vi "Read LINX I2C.vi"(8 "error in (no error)":errorcluster, 11 "TCS3472 in":refnum<class "TCS3472.lvclass">) -> (0 "error out":errorcluster, 2 "LINX I2C":refnum<class "LINX I2C.lvclass">, 3 "TCS3472 out":refnum<class "TCS3472.lvclass">)   [LabVIEW 2020, in "TCS3472.lvclass"]
uses:
  TCS3472.lvclass
  LINX I2C/LINX I2C.lvclass
  TCS3472.lvclass/TCS3472.ctl
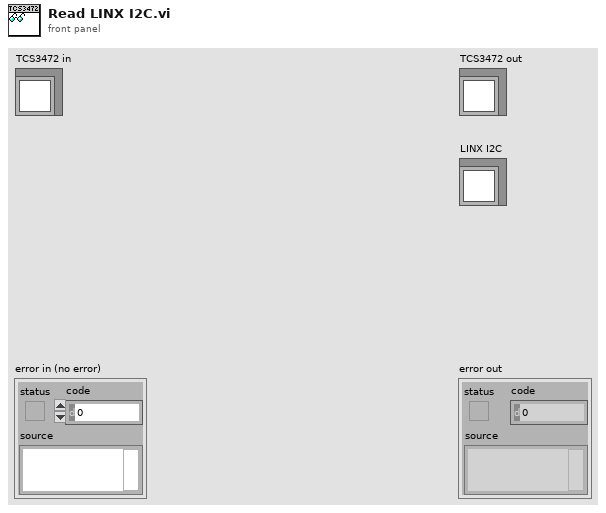
[diagram p1: front panel]
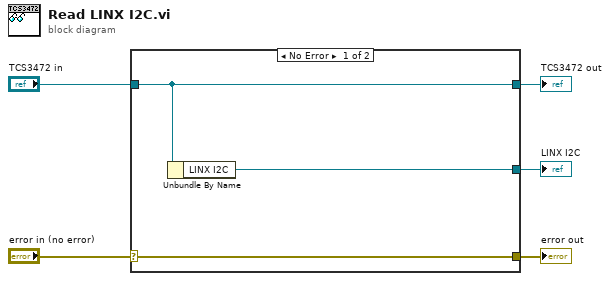
[diagram p0: block diagram]
diagram:
  n1 = case shown="No Error" "error in (no error)" {
    selector: "error in (no error)" -> [w8 w9]
    tunnel: [w8 w9] -> w4
    tunnel: [w7 w10] -> w2
    tunnel: "TCS3472 in" -> [w7 w10]
    tunnel: [w6 _] -> w1
    frame No Error {
      n2 = Unbundle By Name(w7) -> ("LINX I2C"=w6:refnum<class "LINX I2C.lvclass">)
    }
    frame Error {
    }
  }
  "error out" <- w4
  "TCS3472 out" <- w2
  "LINX I2C" <- w1
